vi "Read TDMS.vi"(8 "error in (no error)":errorcluster, 10 "path":path, 11 "LVtoITX in":refnum<class "LVtoITX.lvclass">) -> (0 "error out":errorcluster, 2 "Data":dbl[][](array[numeric]), 3 "Data (Dictionary)":T1[](array[typedef]), 4 "Comments":string, 5 "Wavenames":string[](array[string]), 6 "Igor Commands":string, 7 "LVtoITX out":refnum<class "LVtoITX.lvclass">)   [LabVIEW 2016, in "LVtoITX.lvclass"]
uses:
  LVtoITX.lvclass
  Typedefs/Dictionary--cluster.ctl
  LVtoITX.lvclass/LVtoITX.ctl
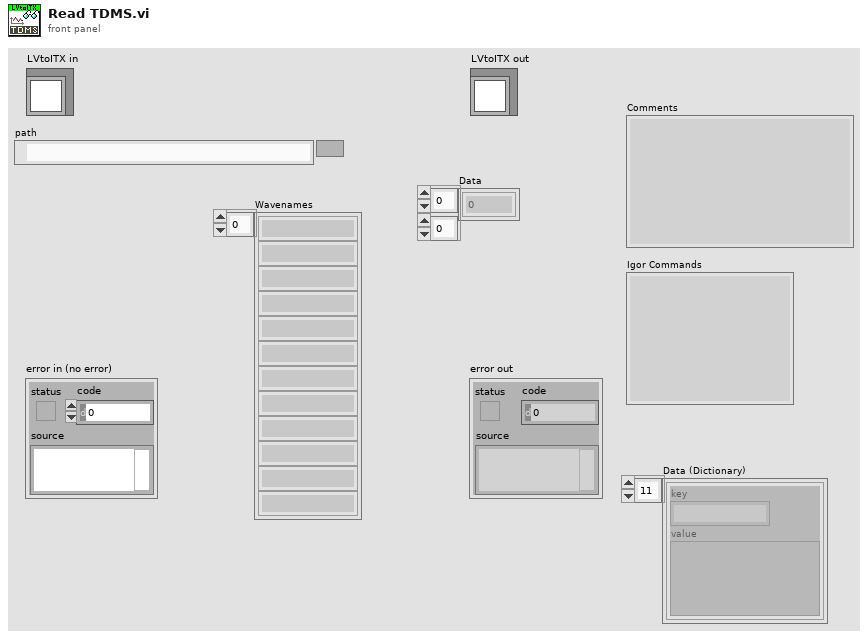
[diagram p1: front panel]
types:
  T1 = typedef "LVtoITX.lvclass/Dictionary--cluster.ctl" = cluster{"key":string, "value":variant}
  T2 = enum16{"open", "open or create", "create or replace", "create", "open (read-only)"}
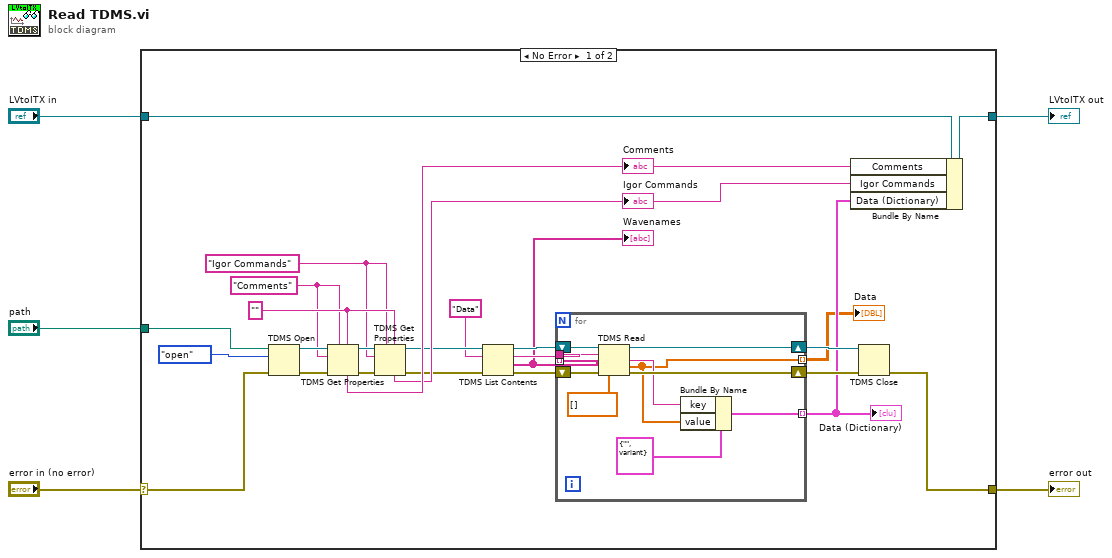
[diagram p0: block diagram]
diagram:
  n1 = case shown="No Error" "error in (no error)" {
    selector: "error in (no error)" -> [w10 w42]
    tunnel: [w19 w42] -> w2
    tunnel: [w30 w43] -> w3
    tunnel: "LVtoITX in" -> [w31 w43]
    tunnel: "path" -> [w9 _]
    frame No Error {
      w26 = "" ("attrib name")
      w13 = "Igor Commands" ("attrib name")
      w14 = "Comments" ("attrib name")
      n2 = TDMS Open(8:w10, 10:T2."open" ("operation (0:open)"), 11:w9) -> (0:w27:errorcluster, 3:w28:refnum<k34>)  [unwired: 4 in]
      n3 = TDMS Get Properties(5:w26, 7:w14, 8:w27, 10:w14, 11:w28) -> (0:w21:errorcluster, 3:w22:refnum<k34>, 4:w25:string)  [unwired: 1 in, 3 out]
      "Comments" <- w25
      n4 = TDMS Get Properties(5:w26, 7:w13, 8:w21, 10:w13, 11:w22) -> (0:w20:errorcluster, 3:w23:refnum<k34>, 4:w24:string)  [unwired: 1 in, 3 out]
      "Igor Commands" <- w24
      n5 = TDMS List Contents(4:w20, 6:"Data" ("group name"), 7:w23) -> (0:w15:errorcluster, 1:w6:string[], 2:w11:string, 3:w17:refnum<k34>)
      "Wavenames" <- w6
      n6 = for {
        shift-right: [w38] -> w16
        shift-left: w15 -> [w41]
        shift-right: [w40] -> w18
        shift-left: w17 -> [w39]
        tunnel: w6 -> [w35] mode=indexing
        tunnel: w11 -> [w36]
        tunnel: [w34] -> w8 mode=indexing
        tunnel: [w32] -> w7 mode=indexing
        n7 = TDMS Read(0:w39, 5:w36, 7:w35, 11:w41, 12:dbl[] [] ("array type (2D Dbl)")) -> (4:w40:refnum<k34>, 10:w32:dbl[], 15:w38:errorcluster)  [unwired: 3 in, 3 out]
        n8 = Bundle By Name(cluster=T1 {"key"="", "value"=variant} ("key-value"), "key"=w35, "value"=w32) -> (w34:T1)
      }
      "Data" <- w7
      "Data (Dictionary)" <- w8
      n9 = Bundle By Name(cluster=w31, "Comments"=w25, "Igor Commands"=w24, "Data (Dictionary)"=w8) -> (w30:refnum<class "LVtoITX.lvclass">)
      n10 = TDMS Close(8:w16, 11:w18) -> (0:w19:errorcluster)  [unwired: 1 out]
    }
    frame Error {
    }
  }
  "error out" <- w2
  "LVtoITX out" <- w3
